vi "Configure Signal_.vi"(7 "Signal Type (0: Voltage)":u16(ring) items=["Voltage", "Current"], 8 "error in (no error)":errorcluster, 9 "Signal Frequency (1000 Hz)":dbl=1000.0, 10 "Signal Level (1.0 V)":dbl=1.0, 11 "Agilent E4980 in":refnum<class "Agilent E4980.lvclass">) -> (0 "error out":errorcluster, 3 "Agilent E4980 out":refnum<class "Agilent E4980.lvclass">)   [LabVIEW 2020, in "Agilent E4980.lvclass"]
uses:
  Agilent E4980.lvclass
  C:/Sandbox/Git_Sandbox/WiSpry Test Framework source code (LV20)/WiSpry Test Framework/Instruments/Instrument.lvclass
  Instrument.lvclass/Instrument.ctl
  Instrument.lvclass
  <instrlib>/Agilent E4980/Agilent E4980.lvlib
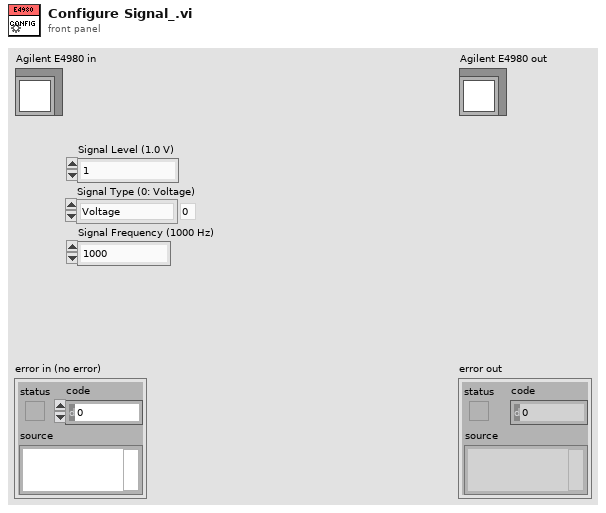
[diagram p1: front panel]
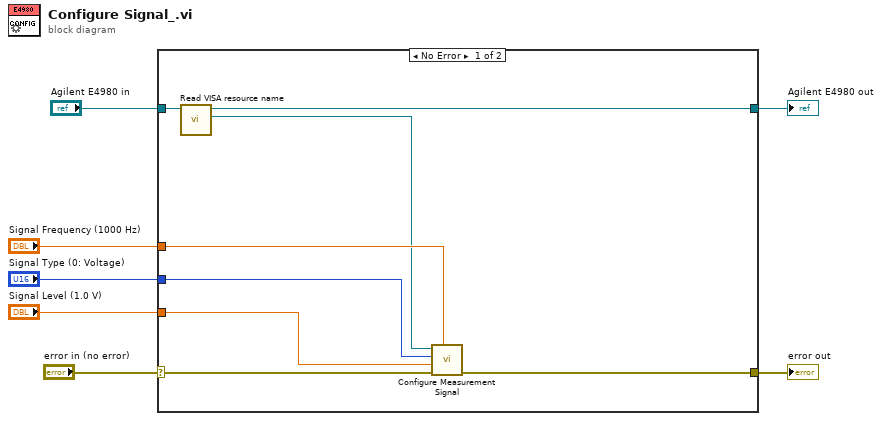
[diagram p0: block diagram]
diagram:
  n1 = case shown="No Error" "error in (no error)" {
    selector: "error in (no error)" -> [w9 w17]
    tunnel: [w8 w17] -> w6
    tunnel: [w14 w16] -> w5
    tunnel: "Agilent E4980 in" -> [w15 w16]
    tunnel: "Signal Frequency (1000 Hz)" -> [w13 _]
    tunnel: "Signal Level (1.0 V)" -> [w12 _]
    tunnel: "Signal Type (0: Voltage)" -> [w11 _]
    frame No Error {
      n2 = call "Read VISA resource name.vi"("Instrument in"=w15) -> ("VISA resource name"=w10:refnum<visa-resource-name>, "Instrument out"=w14:refnum<class "Agilent E4980.lvclass">)  [unwired: 9 in]
      n3 = call <instrlib>:"Configure Measurement Signal.vi"("Signal Frequency (1000 Hz)"=w13, "error in (no error)"=w9, "Signal Level (1.0 V)"=w12, "Signal Type (0: Voltage)"=w11, "VISA resource name"=w10) -> ("error out"=w8:errorcluster)  [unwired: 5 in, 1 out]
    }
    frame Error {
    }
  }
  "error out" <- w6
  "Agilent E4980 out" <- w5
